vi "Indexer Controller.vi"(8 "error in":errorcluster) -> ()   [LabVIEW 2019]
doc: "This VI executes continuously carrying out the current operation and responding to updates or new operations. It will often contain the timing or control code that is difficult to place directly in TeleOp. This VI generally opens all sensors and motors and isolates the rest of the robot code from knowing how the operations are carried out."
uses:
  Indexer Operations.ctl
  Indexer Setpoints.ctl
  <vilib>/Rock Robotics/Network Tables/NT Write Boolean.vi
  <vilib>/Rock Robotics/WPI/Framework/Completion Status.ctl
panel:
  in  "Interactive Values":T1
  out "Current\nCmd":string
  in  "Buttons":cluster{"Execute Cmd":bool, "Abort Cmd":bool}
  out "Command Timing":cluster{"Start Time (ms)":u32, "Iterations":i32}
  out "Status":T3
  # "Tip: It may be helpful to observe inputs and sensor values.\nYou may also want to display tuning or debugging controls."
  # "Interactive Command: You may fill in the settings for a command\nand schedule it with the Execute button. You can observe and abort\nany command while fine tuning the code for the controller."
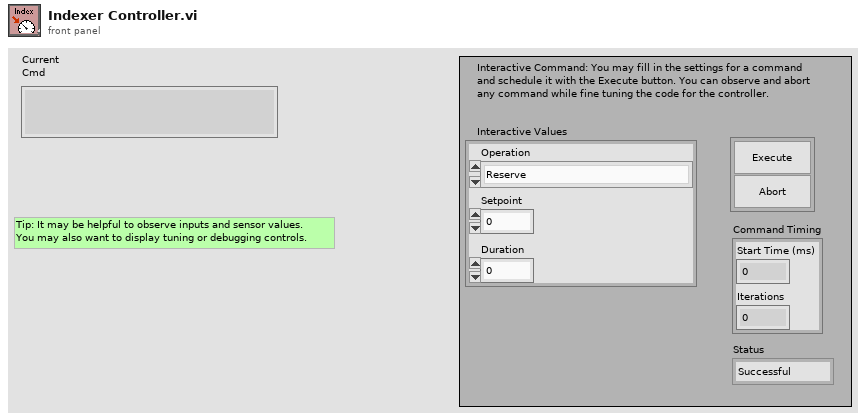
[diagram p1: front panel]
types:
  T1 = typedef "Indexer Setpoints.ctl" = cluster{"Operation":T2, "Setpoint":dbl, "Duration":dbl}
  T2 = typedef "Indexer Operations.ctl" = enum16{"Reserve", "Read Current", "Immediate", "Index", "ReverseIndex"}
  T3 = typedef "Completion Status.ctl" = enum16{"Successful", "Aborted", "Incomplete"}
  T4 = typedef "WPI_MotorControlDeviceRef.ctl" = cluster{"DeviceStatus":errorcluster, "Type":T5, "PWM":cluster{"PWM Channel":T6, "DeadBand":T7}, "CAN":cluster{"Device Number":u8, "SetOutput VI Ref":variant, "GetOutput VI Ref":variant, "Enable VI Ref":variant, "Disable VI Ref":variant, "Data":variant}, "Invert":bool, "DIO PWM":cluster{"PWM \"Enable\" Channel":T6, "DIOChannel":T8, "PWM Rate":dbl}}
  T5 = typedef "WPI_MotorControlType.ctl" = enum16{"PWM", "CAN", "DIO PWM"}
  T6 = typedef "FPGA_DIOPWMChannel.ctl" = enum8{"PWM 0", "PWM 1", "PWM 2", "PWM 3", "PWM 4", "PWM 5", "PWM 6", "PWM 7", "PWM 8", "PWM 9", "PWM MXP 0", "PWM MXP 1", "PWM MXP 2", "PWM MXP 3", "PWM MXP 4", "PWM MXP 5", "PWM MXP 6", "PWM MXP 7", "PWM MXP 8", "PWM MXP 9", "Invalid"}
  T7 = typedef "WPI_PWMDeadband.ctl" = cluster{"Name":string, "maxPositivePwm":i32, "minPositivePwm":i32, "centerPwm":i32, "maxNegativePwm":i32, "minNegativePwm":i32, "angularRange":u16}
  T8 = typedef "FPGA_DIOChannel.ctl" = enum8{"DIO 0", "DIO 1", "DIO 2", "DIO 3", "DIO 4", "DIO 5", "DIO 6", "DIO 7", "DIO 8", "DIO 9", "DIO MXP 0", "DIO MXP 1", "DIO MXP 2", "DIO MXP 3", "DIO MXP 4", "DIO MXP 5", "DIO MXP 6", "DIO MXP 7", "DIO MXP 8", "DIO MXP 9", "DIO MXP 10", "DIO MXP 11", "DIO MXP 12", "DIO MXP 13", "DIO MXP 14", "DIO MXP 15", "SPI Port CS1", "SPI Port CS2", "SPI Port CS3", "SPI Port MISO", "SPI Port MOSI", "Invalid"}
  T9 = typedef "Command Status Info.ctl" = cluster{"Name":string, "Status":T3, "notifier out":T10}
  T10 = typedef "Completion Notifier.ctl" = refnum<notifier>
  T11 = cluster{"Current Command":T1, "Command Timing":cluster{"Start Time (ms)":u32, "Iterations":i32}, "Command Arguments":cluster{"Command Info":T9, "Description":string, "Default Command":T1, "queue out":refnum<queue>, "Subsystem Name":string}}
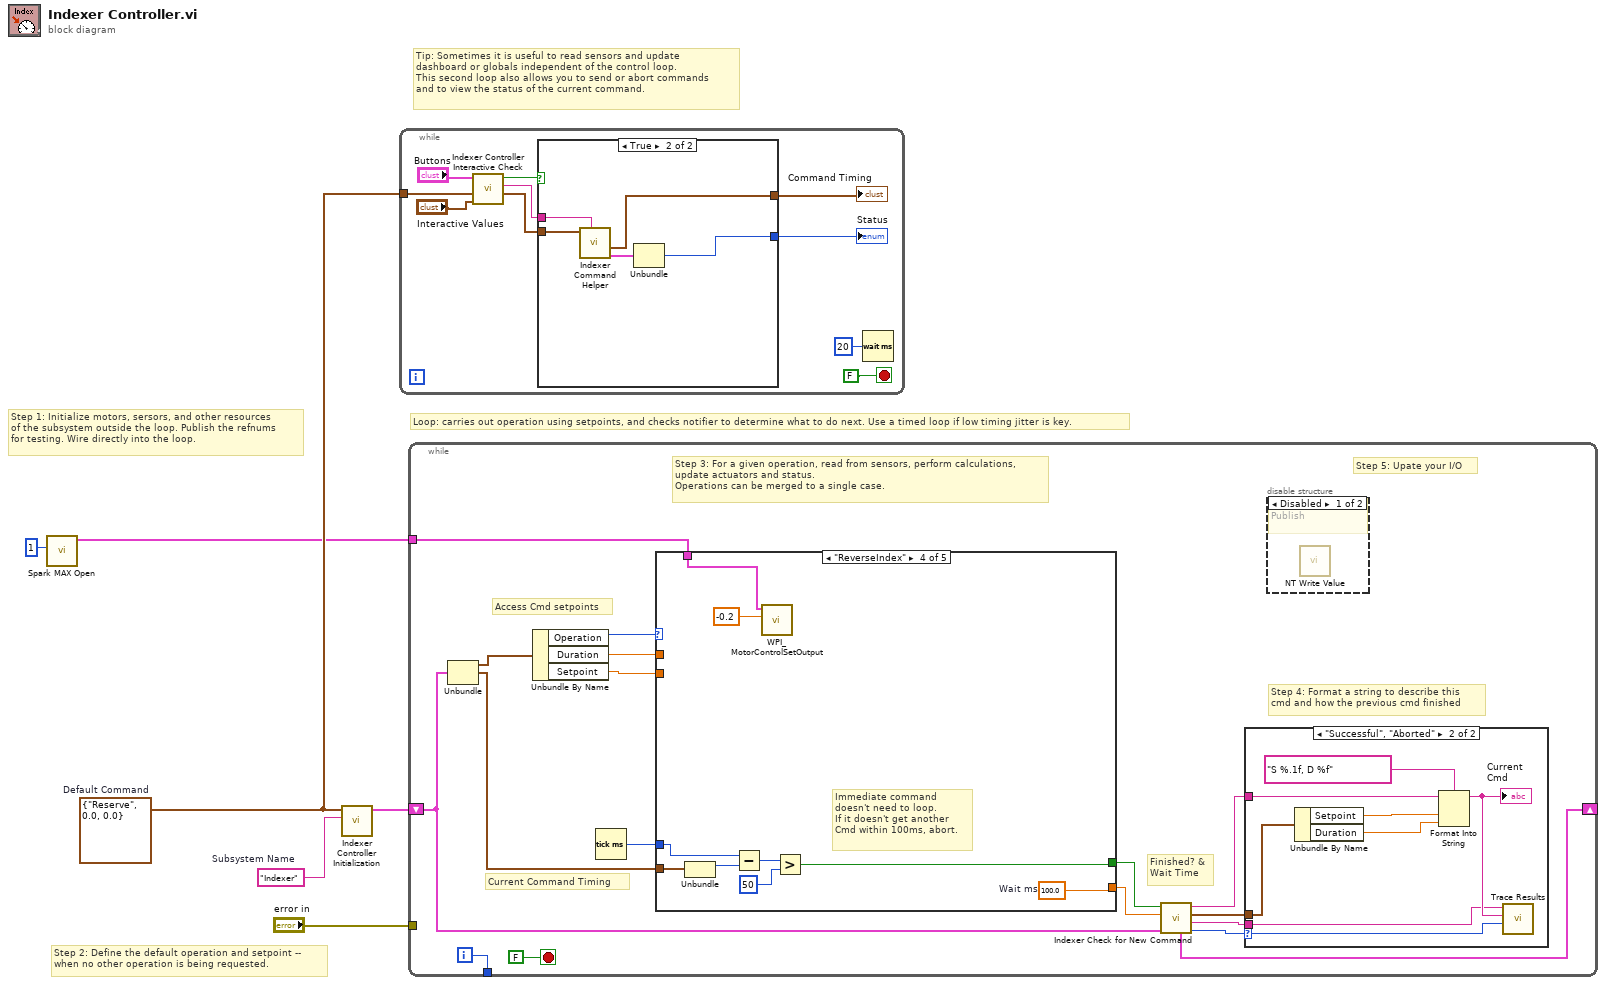
[diagram p0: block diagram]
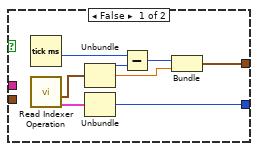
[diagram p2: hidden frame]
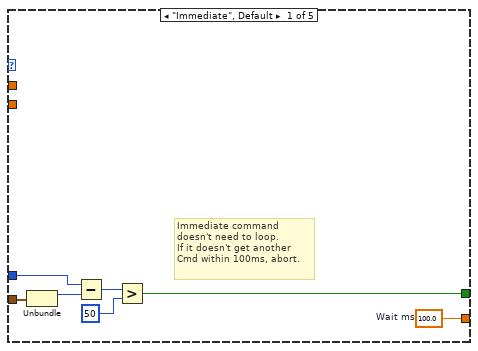
[diagram p5: hidden frame]
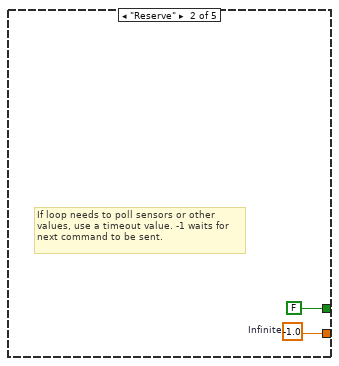
[diagram p6: hidden frame]
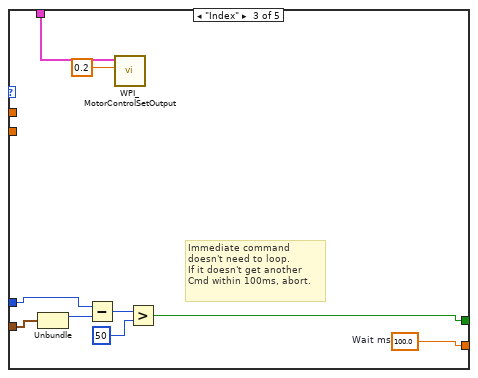
[diagram p7: hidden frame]
diagram:
  w3 = T1 {"Operation"=enum."Reserve", "Setpoint"=0.0, "Duration"=0.0}  # Default Command
  w4 = "Indexer"  # Subsystem Name
  # "Tip: Sometimes it is useful to read sensors and update\ndashboard or globals independent of the control loop.\nThis second loop also allows you to send or abort commands\nand to view the status of the current command."
  # "Step 2: Define the default operation and setpoint --\nwhen no other operation is being requested."
  # "Step 1: Initialize motors, sersors, and other resources\nof the subsystem outside the loop. Publish the refnums\nfor testing. Wire directly into the loop."
  # "Loop: carries out operation using setpoints, and checks notifier to determine what to do next. Use a timed loop if low timing jitter is key."
  n1 = call <vilib>:"Spark MAX Open.vi"("Device Number"=u8 1) -> ("MotorControlDeviceRef"=w1:T4)  [unwired: 9 in, 1 out]
  n2 = call "Indexer Controller Initialization.vi"("Subsystem Name"=w4, "Default Command"=w3) -> ("Current Command"=w5:T11)  [unwired: 9 in]
  n3 = while {
    tunnel: w3 -> [w13]
    stop <- FALSE stop-if-true
    n4 = call "Indexer Controller Interactive Check.vi"("Interactive Command in"="Interactive Values", "Default Command"=w13, "Buttons"="Buttons") -> ("Interactive Command out"=w10:T1, "Trace String"=w11:string, "Schedule"=w12:bool)  [unwired: 6 in]
    n5 = case shown="True" w12 {
      tunnel: [w24 w29] -> w9
      tunnel: w10 -> [_ w27]
      tunnel: [w20 w25] -> w8
      tunnel: w11 -> [_ w28]
      frame False {
        n6 = Tick Count (ms)() -> (millisecond timer value=w19:u32)
        n7 = call "Read Indexer Operation.vi"() -> ("Command Info"=w17:T9, "SubSystem Data"=w18:T1)  [unwired: 9 in, 1 out]
        n8 = Unbundle(w18) -> ("Operation"=w23:T2, "Setpoint"=w21:dbl)  [unwired: 1 out]
        n9 = Unbundle(w17) -> ("Status"=w24:T3)  [unwired: 2 out]
        n10 = Subtract(x=w19, y=w23) -> (x-y=w22:u32)
        n11 = Bundle(w22, "Setpoint"=w21) -> (w20:cluster{u32, "Setpoint":dbl})  [unwired: 1 in]
      }
      frame True {
        n12 = call "Indexer Command Helper.vi"("Description"=w28, "SubSystem Data"=w27) -> ("Command Info Out"=w26:T9, "Command Timing"=w25:cluster{"Start Time (ms)":u32, "Iterations":i32})  [unwired: 7 in, 1 out]
        n13 = Unbundle(w26) -> ("Status"=w29:T3)  [unwired: 2 out]
      }
    }
    "Status" <- w9
    "Command Timing" <- w8
    n14 = Wait (ms)(milliseconds to wait=u32 20) -> ()  [unwired: 1 out]
  }
  n15 = while {
    shift-right: [w38] -> _
    shift-left: w5 -> [w31]
    tunnel: [w45] -> _
    tunnel: "error in" -> [_]
    tunnel: w1 -> [w30]
    i -> [w45]
    stop <- FALSE stop-if-true
    # "Step 5: Upate your I/O"
    # "Step 4: Format a string to describe this\ncmd and how the previous cmd finished"
    # "Current Command Timing"
    # "Access Cmd setpoints"
    # "Finished? &\nWait Time"
    # "Step 3: For a given operation, read from sensors, perform calculations,\nupdate actuators and status.\nOperations can be merged to a single case."
    n16 = Unbundle(w31) -> ("Current Command"=w44:T1, "Command Timing"=w40:cluster{"Start Time (ms)":u32, "Iterations":i32})  [unwired: 1 out]
    n17 = Unbundle By Name(w44) -> ("Operation"=w43:T2, "Duration"=w42:dbl, "Setpoint"=w39:dbl)
    n18 = Tick Count (ms)() -> (millisecond timer value=w41:u32)
    n19 = case shown="\"ReverseIndex\"" w43 {
      tunnel: [w61 w63 w64 w75 _] -> w36
      tunnel: [w55 FALSE ("ignore previous (F)") w67 w73 _] -> w37
      tunnel: w40 -> [w57 _ w66 w76 _]
      tunnel: w42 -> [_ _ _ _ _]
      tunnel: w41 -> [w56 _ w65 w77 _]
      tunnel: w39 -> [_ _ _ _ _]
      tunnel: w30 -> [_ _ w72 w74 _]
      frame "Immediate", Default {
        w61 = 100.0  # Wait ms
        # "Immediate command\ndoesn't need to loop.\nIf it doesn't get another\nCmd within 100ms, abort."
        n20 = Unbundle(w57) -> ("Start Time (ms)"=w60:u32)  [unwired: 1 out]
        n21 = Subtract(x=w56, y=w60) -> (x-y=w59:u32)
        n22 = Greater?(x=w59, y=u8 50 ("Left Motor")) -> (0:w55:bool)
      }
      frame "Reserve" {
        w63 = -1.0  # Infinite
        # "If loop needs to poll sensors or other\nvalues, use a timeout value. -1 waits for\nnext command to be sent."
      }
      frame "Index" {
        w64 = 100.0  # Wait ms
        # "Immediate command\ndoesn't need to loop.\nIf it doesn't get another\nCmd within 100ms, abort."
        n23 = Unbundle(w66) -> ("Start Time (ms)"=w70:u32)  [unwired: 1 out]
        n24 = Subtract(x=w65, y=w70) -> (x-y=w69:u32)
        n25 = call <vilib>:"WPI_MotorControlSetOutput.vi"("Output"=0.2 ("Motor Output"), "MotorControlDevRef"=w72) -> ()  [unwired: 7 in, 3 out]
        n26 = Greater?(x=w69, y=u8 50 ("Left Motor")) -> (0:w67:bool)
      }
      frame "ReverseIndex" {
        w75 = 100.0  # Wait ms
        # "Immediate command\ndoesn't need to loop.\nIf it doesn't get another\nCmd within 100ms, abort."
        n27 = Unbundle(w76) -> ("Start Time (ms)"=w80:u32)  [unwired: 1 out]
        n28 = Subtract(x=w77, y=w80) -> (x-y=w79:u32)
        n29 = call <vilib>:"WPI_MotorControlSetOutput.vi"("Output"=-0.2 ("Motor Output"), "MotorControlDevRef"=w74) -> ()  [unwired: 7 in, 3 out]
        n30 = Greater?(x=w79, y=u8 50 ("Left Motor")) -> (0:w73:bool)
      }
      frame "Read Current" {
      }
    }
    n31 = call "Indexer Check for New Command.vi"("Current Command"=w31, "Wait time (ms)"=w36, "Finished?"=w37) -> ("Completion"=w32:T3, "Subsystem Name"=w33:string, "Current Command"=w34:T1, "Initial Trace String"=w35:string, "NextCommand"=w38:T11)  [unwired: 4 in]
    n32 = case shown="\"Successful\", \"Aborted\"" w32 {
      selector: w32 -> [_ w54]
      tunnel: w35 -> [_ w50]
      tunnel: w34 -> [_ w51]
      tunnel: w33 -> [_ w47]
      frame "Incomplete", Default {
        # "Continuing current command"
      }
      frame "Successful", "Aborted" {
        # "Report and setup for next command"
        n33 = Unbundle By Name(w51) -> ("Setpoint"=w53:dbl, "Duration"=w48:dbl)
        n34 = Format Into String(format string="S %.1f, D %f", initial string=w50, w53, w48) -> (resulting string=w49:string)  [unwired: 1 in, 1 out]
        "Current\nCmd" <- w49
        n35 = call <vilib>:"Trace Results.vi"("Status of previous command"=w54, "Description"=w49, "Subsystem"=w47) -> ()  [unwired: 9 in]
      }
    }
    n36 = disable-structure shown="Disabled" {
      frame Disabled {
        # "Publish"
        n37 = call-poly <vilib>:"NT Write Value.vi"() -> ()  [unwired: 11 in, 1 out]
      }
      frame Enabled {
      }
    }
  }
